vi "PixelsToVolts4.vi"(2 "Last Mouse Position":cluster{"X":i32, "Y":i32}, 3 "Calibration \nCoordinates":T1) -> (0 "Y in volts":sgl, 1 "X in volts":sgl)   [LabVIEW 2011]
uses:
  <vilib>/Analysis/baseanly.llb/Real Inverse Matrix.vi
  <vilib>/Analysis/Matrix/Numeric/Multiply/Multiply - RM,RM.vi
  <vilib>/Analysis/NI_AALBase.lvlib
  <vilib>/Analysis/Matrix/NI_Matrix.lvlib
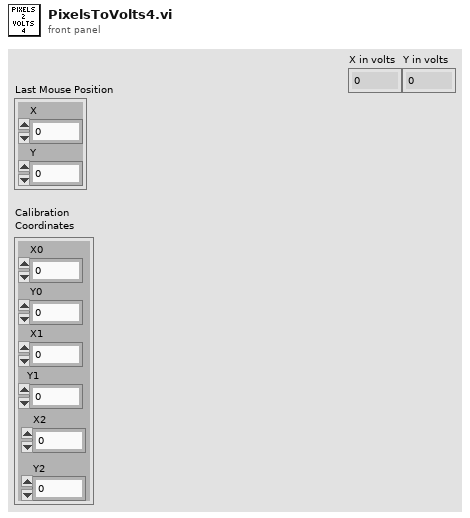
[diagram p1: front panel]
types:
  T1 = cluster{"X0":sgl, "Y0":sgl, "X1":sgl, "Y1":sgl, "X2":dbl, "Y2":dbl}
  T2 = typedef "NI_Matrix.lvlib/RealMatrix.ctl" = dbl[][]
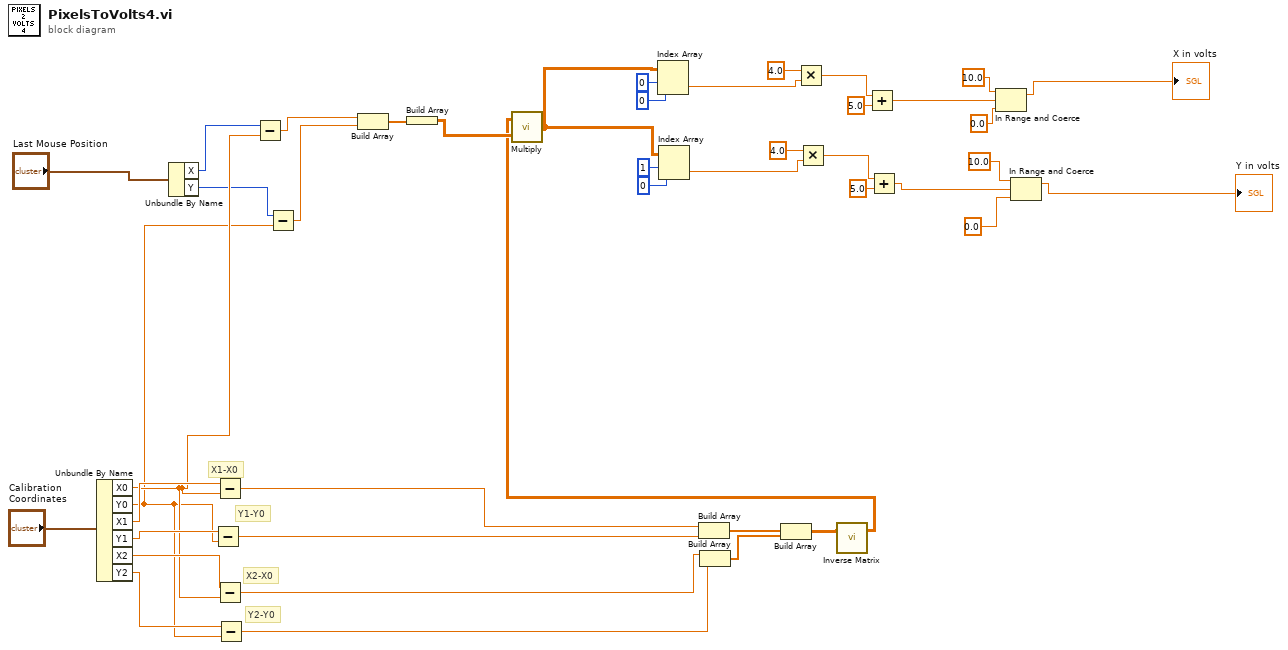
[diagram p0: block diagram]
diagram:
  # "Y2-Y0"
  # "X2-X0"
  # "Y1-Y0"
  # "X1-X0"
  n1 = Unbundle By Name("Calibration \nCoordinates") -> ("X0"=w25:sgl, "Y0"=w23:sgl, "X1"=w35:sgl, "Y1"=w33:sgl, "X2"=w34:dbl, "Y2"=w32:dbl)
  n2 = Unbundle By Name("Last Mouse Position") -> ("X"=w24:i32, "Y"=w22:i32)
  n3 = Subtract(x=w33, y=w23) -> (x-y=w30:sgl)
  n4 = Subtract(x=w35, y=w25) -> (x-y=w31:sgl)
  n5 = Subtract(x=w34, y=w25) -> (x-y=w29:dbl)
  n6 = Subtract(x=w32, y=w23) -> (x-y=w28:dbl)
  n7 = Subtract(x=w24, y=w25) -> (x-y=w21:sgl)
  n8 = Subtract(x=w22, y=w23) -> (x-y=w20:sgl)
  n9 = Build Array(w21, w20) -> (w17:sgl[])
  n10 = Build Array(w17) -> (w19:T2)
  n11 = Build Array(w31, w30) -> (w27:sgl[])
  n12 = Build Array(w29, w28) -> (w26:dbl[])
  n13 = Build Array(w27, w26) -> (w18:T2)
  n14 = call-poly <vilib>:"Inverse Matrix.vi"("Input Matrix"=w18) -> ("Inverse Matrix"=w16:T2)  [unwired: 1 in, 1 out]
  n15 = call-poly <vilib>:"Multiply.vi"("Real Matrix B"=w19, "Real Matrix A"=w16) -> ("A * B"=w11:T2)
  n16 = Index Array(array=w11, index (row)=0, index (col)=0) -> (element=w2:dbl)
  n17 = Index Array(array=w11, index (row)=1, index (col)=0) -> (element=w1:dbl)
  n18 = Multiply(x=4.0, y=w2) -> (x*y=w6:dbl)
  n19 = Multiply(x=4.0, y=w1) -> (x*y=w5:dbl)
  n20 = Add(x=w6, y=5.0) -> (x+y=w4:dbl)
  n21 = Add(x=w5, y=5.0) -> (x+y=w3:dbl)
  n22 = In Range and Coerce(upper limit=10.0, x=w4, lower limit=0.0) -> (coerced(x)=→"X in volts":dbl)  [unwired: 1 out]
  n23 = In Range and Coerce(upper limit=10.0, x=w3, lower limit=0.0) -> (coerced(x)=→"Y in volts":dbl)  [unwired: 1 out]
